vi "Create.vi"(8 "error in (no error)":errorcluster, 10 "WebView2 Control Ref":refnum<vi>, 11 "Type":refnum<class "WebView2 QControl.lvclass">) -> (0 "error out":errorcluster, 3 "WebView2 Control out":refnum<class "WebView2 QControl.lvclass">)   [LabVIEW 2020, in "WebView2 QControl.lvlib" / "WebView2 QControl.lvclass"]
uses:
  WebView2 QControl.lvclass
  Webview2 Lib/WebView2 Control Object/WebView2 Control.lvclass
  WebView2 QControl.lvclass/WebView2 QControl.ctl
  C:/Users/Simon/Documents/GitHub/LV-WebView2/Source/Libs/Microsoft.Web.WebView2.WinForms.dll
  Libs/Microsoft.Web.WebView2.WinForms.dll
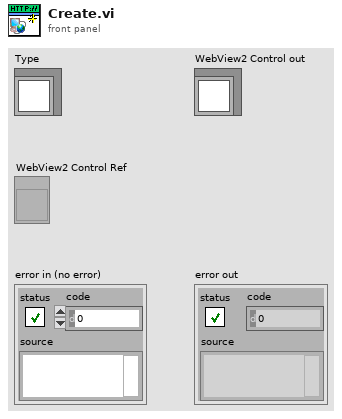
[diagram p1: front panel]
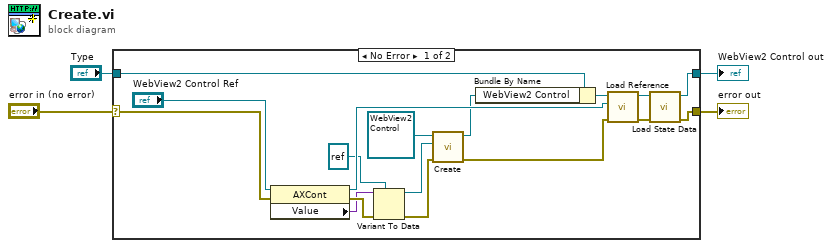
[diagram p0: block diagram]
diagram:
  n1 = case shown="No Error" "error in (no error)" {
    selector: "error in (no error)" -> [w20 w23]
    tunnel: [w7 w23] -> w3
    tunnel: [w5 w22] -> w1
    tunnel: "Type" -> [w21 w22]
    frame No Error {
      n2 = property class="AXCont"(reference="WebView2 Control Ref", error in=w20) -> (reference out=w16:refnum<vi>, error out=w18:errorcluster, "Value"=w15:variant)
      n3 = Variant To Data(error in=w18, type=refnum<k24> refnum ("WebView2 Control"), Variant=w15) -> (data=w9:refnum<k24>, error out=w12:errorcluster)
      n4 = call "Create.vi"("error in (no error)"=w12, "WebView2 Control"=w9, "Type"=refnum<class "WebView2 Control.lvclass"> refnum ("Control Type")) -> ("error out"=w11:errorcluster, "WebView2 Control out"=w10:refnum<class "WebView2 Control.lvclass">)  [unwired: 7 in]
      n5 = Bundle By Name(cluster=w21, "WebView2 Control"=w10) -> (w13:refnum<class "WebView2 QControl.lvclass">)
      n6 = call-dynamic "Load Reference.vi"("error in (no error)"=w11, "Reference"=w16, "ActiveX Control in"=w13) -> ("error out"=w19:errorcluster, "ActiveX Control out"=w6:refnum<class "WebView2 QControl.lvclass">)  [unwired: 7 in]
      n7 = call-dynamic "Load State Data.vi"("error in (no error)"=w19, "Control in"=w6) -> ("error out"=w7:errorcluster, "Control out"=w5:refnum<class "WebView2 QControl.lvclass">)  [unwired: 8 in]
    }
    frame Error {
    }
  }
  "error out" <- w3
  "WebView2 Control out" <- w1
